vi "RTM SLSC Autodetect.vi"(8 "error in (no error)":errorcluster, 11 "Node Ptr":T1=18446744073709551615 format="%.0x") -> (0 "error out":errorcluster)   [LabVIEW 2017, in "SLSC EDS System Explorer.lvlib"]
uses:
  SLSC EDS System Explorer.lvlib
  <vilib>/NI Veristand/Custom Device API/Custom Device Item Ref.ctl
  <vilib>/NI VeriStand/Custom Device Tools/Custom Device Utility Library/Custom Device Utility Library.lvlib
  <vilib>/NI VeriStand/Custom Device API/Custom Device API.lvlib
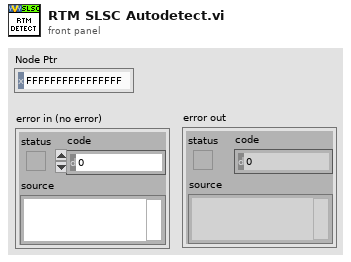
[diagram p1: front panel]
types:
  T1 = typedef "Custom Device API.lvlib/Custom Device Item Ref.ctl" = u64
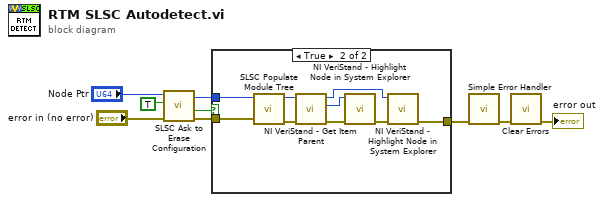
[diagram p0: block diagram]
diagram:
  n1 = call "SLSC Ask to Erase Configuration.vi"("error in (no error)"="error in (no error)", "Ask to erase?"=TRUE, "Device Item Ref in"="Node Ptr") -> ("error out"=w3:errorcluster, "Erase Data?"=w2:bool, "Item Ref out"=w1:T1)  [unwired: 5 in, 1 out]
  n2 = case shown="True" w2 {
    tunnel: [w10 w14] -> w7
    tunnel: w3 -> [w10 w12]
    tunnel: w1 -> [_ w11]
    frame False {
    }
    frame True {
      n3 = call "SLSC Populate Module Tree.vi"("error in (no error)"=w12, "Device Item Ref in"=w11) -> ("error out"=w18:errorcluster, "Device Item Ref out"=w19:T1)  [unwired: 5 in, 3 out]
      n4 = call <vilib>:"NI VeriStand - Get Item Parent.vi"("error in (no error)"=w18, "Item Ref in"=w19) -> ("error out"=w16:errorcluster, "Parent Ref"=w13:T1, "Item Ref out"=w17:T1)  [unwired: 6 in, 1 out]
      n5 = call <vilib>:"NI VeriStand - Highlight Node in System Explorer.vi"("error in (no error)"=w16, "Item Ref in"=w13) -> ("error out"=w15:errorcluster)  [unwired: 8 in, 1 out]
      n6 = call <vilib>:"NI VeriStand - Highlight Node in System Explorer.vi"("error in (no error)"=w15, "Item Ref in"=w17) -> ("error out"=w14:errorcluster)  [unwired: 8 in, 1 out]
    }
  }
  n7 = call <vilib>:"Simple Error Handler.vi"("error in (no error)"=w7) -> ("error out"=w9:errorcluster)  [unwired: 4 in, 4 out]
  n8 = call <vilib>:"Clear Errors.vi"("error in (no error)"=w9) -> ("error out"=→"error out":errorcluster)  [unwired: 5 in, 1 out]
